vi "IR_Correction_test.vi"() -> ()   [LabVIEW 2019]
uses:
  WSCbot_V3_Toolkit.lvlibp/WSCBOTV3_Toolkit/Sensor/LowLevel/IR_Chanel.ctl
  WSCbot_V3_Toolkit.lvlibp
panel:
  out "cluster":T1
  out "Valtage":dbl[](array[numeric])
  in  "Stop Button":bool
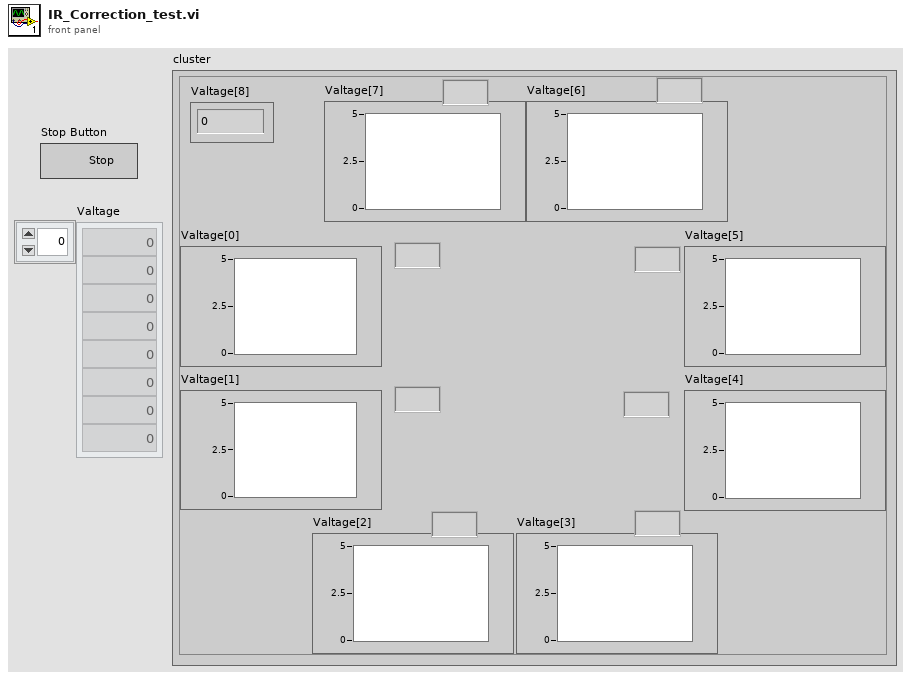
[diagram p1: front panel]
types:
  T1 = cluster{"Valtage[0]":dbl, "Valtage[1]":dbl, "Valtage[2]":dbl, "Valtage[3]":dbl, "Valtage[4]":dbl, "Valtage[5]":dbl, "Valtage[6]":dbl, "Valtage[7]":dbl, "Valtage[8]":dbl}
  T2 = typedef "WSCbot_V3_Toolkit.lvlibp/IR_Chanel.ctl" = enum16{"IR_LF", "IR_LB", "IR_BL", "IR_BR", "IR_RB", "IR_RF", "IR_FR", "IR_FL"}
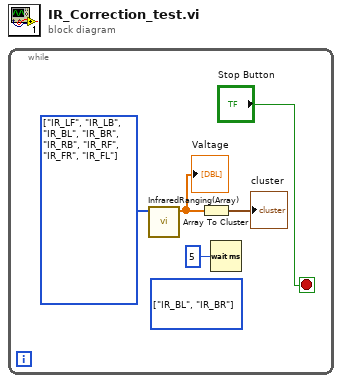
[diagram p0: block diagram]
diagram:
  n1 = while {
    stop <- "Stop Button" stop-if-true
    (unwired) T2[] [enum."IR_BL", enum."IR_BR"] items=["IR_LF", "IR_LB", "IR_BL", "IR_BR", "IR_RB", "IR_RF", "IR_FR", "IR_FL"] ("IR_Chanel")
    w5 = T2[] [enum."IR_LF", enum."IR_LB", enum."IR_BL", enum."IR_BR", enum."IR_RB", enum."IR_RF", enum."IR_FR", enum."IR_FL"] items=["IR_LF", "IR_LB", "IR_BL", "IR_BR", "IR_RB", "IR_RF", "IR_FR", "IR_FL"] ("IR_Chanel")
    n2 = call "InfraredRanging(Array).vi"("IR_Chanel"=w5) -> ("Valtage"=w3:dbl[])  [unwired: 9 in, 1 out]
    "Valtage" <- w3
    n3 = Array To Cluster(array=w3) -> (cluster=→"cluster":T1)
    n4 = Wait (ms)(milliseconds to wait=u32 5) -> ()  [unwired: 1 out]
  }
